vi "shift regester.vi"() -> ()   [LabVIEW 2025]
panel:
  out "Numeric 3":dbl
  out "Boolean":bool
  out "Numeric 2":dbl
  out "Numeric":dbl
  out "o/p":dbl
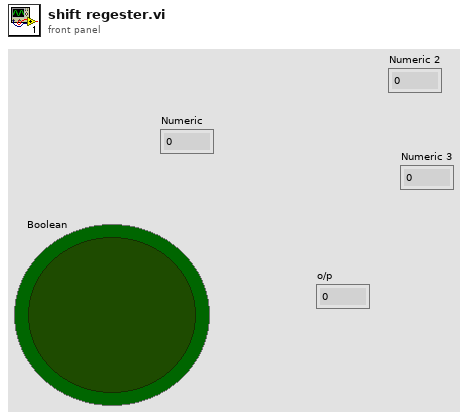
[diagram p1: front panel]
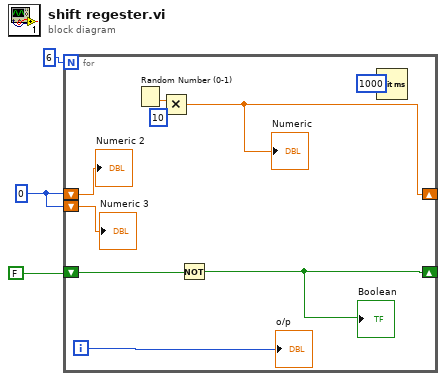
[diagram p0: block diagram]
diagram:
  w1 = 0
  n1 = for {
    N: 6 -> [_]
    shift-right: [w8] -> _
    shift-left: w1 -> [w7]
    shift-right: [w5] -> _
    shift-left: FALSE -> [w6]
    shift-left: w1 -> [w4]
    i -> [w12]
    n2 = Random Number (0-1)() -> (number: 0 to 1=w10:dbl)
    n3 = Multiply(x=w10, y=10) -> (x*y=w8:dbl)
    "Numeric" <- w8
    n4 = Not(x=w6) -> (.not. x?=w5:bool)
    "Boolean" <- w5
    n5 = Wait (ms)(milliseconds to wait=1000) -> ()  [unwired: 1 out]
    "o/p" <- w12
    "Numeric 2" <- w7
    "Numeric 3" <- w4
  }
